vi "模拟反馈.vi"(0 "拆分信息-数据":T2, 5 "寄存器输入":u16[](array[numeric])) -> (14 "反馈参数":T1, 19 "寄存器输出":u16[](array[numeric]))   [LabVIEW 2019, in "MainPage.lvlib" / "MainPage.lvclass"]
uses:
  MainPage.lvclass
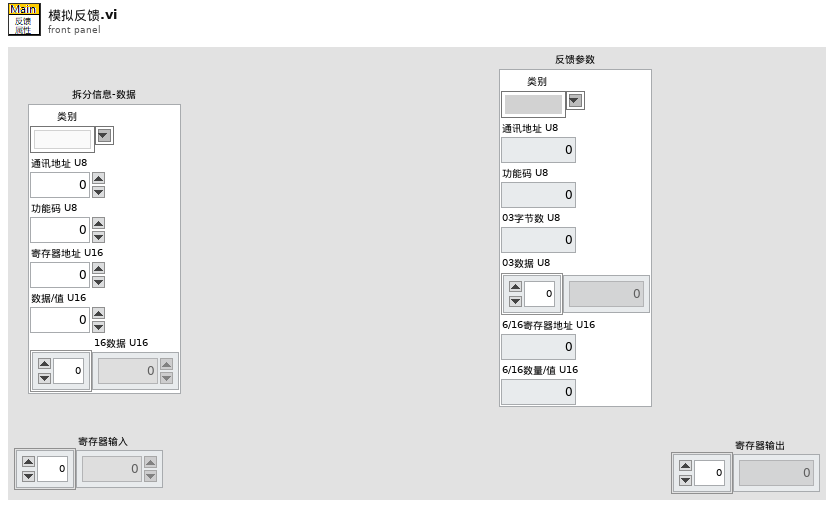
[diagram p1: front panel]
types:
  T1 = cluster{"类别":string, "通讯地址 U8":u8, "功能码 U8":u8, "03字节数 U8":u8, "03数据 U8":u8[], "6/16寄存器地址 U16":u16, "6/16数量/值 U16":u16}
  T2 = cluster{"类别":string, "通讯地址 U8":u8, "功能码 U8":u8, "寄存器地址 U16":u16, "数据/值 U16":u16, "16数据 U16":u16[]}
  T3 = cluster{"类别":string, "通讯地址 U8":u8, "功能码 U8":u8, u8, u8[], "寄存器地址 U16":u16, "数据/值 U16":u16}
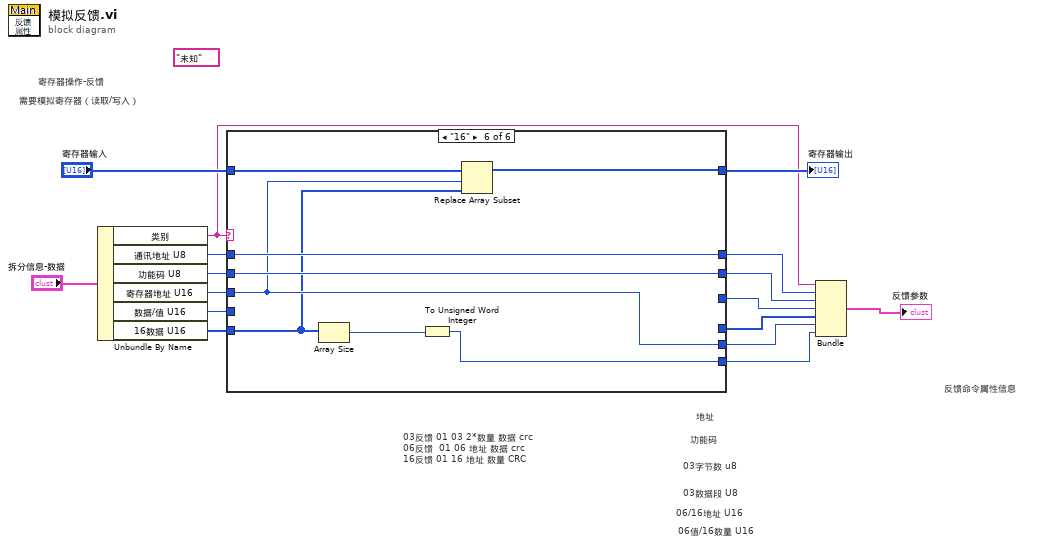
[diagram p0: block diagram]
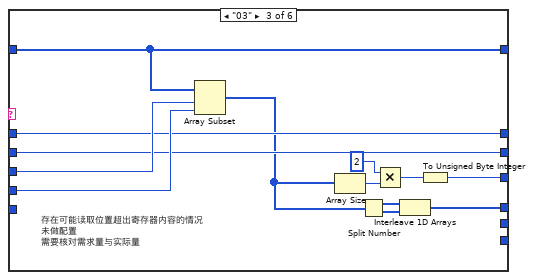
[diagram p4: hidden frame]
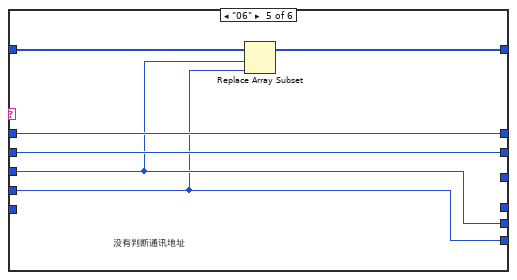
[diagram p6: hidden frame]
diagram:
  (unwired) "未知" ("类别")
  # "06值/16数量 U16"
  # "06/16地址 U16"
  # "03数据段 U8"
  # "03字节数 u8"
  # "功能码"
  # "地址"
  # "03反馈 01 03 2*数量 数据 crc\n06反馈  01 06 地址 数据 crc\n16反馈 01 16 地址 数量 CRC"
  # "反馈命令属性信息"
  # "需要模拟寄存器（读取/写入）"
  # "寄存器操作-反馈"
  n1 = Unbundle By Name("拆分信息-数据") -> ("类别"=w1:string, "通讯地址 U8"=w13:u8, "功能码 U8"=w12:u8, "寄存器地址 U16"=w11:u16, "数据/值 U16"=w10:u16, "16数据 U16"=w9:u16[])
  n2 = case shown="\"16\"" w1 {
    tunnel: "寄存器输入" -> [w17 w18 w31 w32 w36 w46]
    tunnel: [w17 w18 w31 w32 w33 w45] -> w14
    tunnel: w13 -> [_ _ w28 _ w38 w44]
    tunnel: w12 -> [_ _ w27 _ w37 w43]
    tunnel: w11 -> [_ _ w30 _ w35 w41]
    tunnel: w10 -> [_ _ w29 _ w34 _]
    tunnel: w9 -> [_ _ _ _ _ w40]
    tunnel: [_ _ w28 _ w38 w44] -> w8
    tunnel: [_ _ w27 _ w37 w43] -> w7
    tunnel: [_ _ w20 _ _ _] -> w5
    tunnel: [_ _ w19 _ _ _] -> w6
    tunnel: [_ _ _ _ w35 w41] -> w4
    tunnel: [_ _ _ _ w34 w42] -> w3
    frame Default {
    }
    frame "未知" {
    }
    frame "03" {
      # "存在可能读取位置超出寄存器内容的情况\n未做配置\n需要核对需求量与实际量"
      n3 = Array Subset(array=w31, index=w30, length=w29) -> (w21:u16[])
      n4 = Array Size(array=w21) -> (size(s)=w26:i32)
      n5 = Split Number(x=w21) -> (hi(x)=w23:u8[], lo(x)=w22:u8[])
      n6 = Multiply(x=2, y=w26) -> (x*y=w24:i32)
      n7 = Interleave 1D Arrays(w23, w22) -> (w20:u8[])
      n8 = To Unsigned Byte Integer(number=w24) -> (unsigned 8bit integer=w19:u8)
    }
    frame "05" {
    }
    frame "06" {
      # "没有判断通讯地址"
      n9 = Replace Array Subset(array=w36, new element=w34, index=w35) -> (w33:u16[])
    }
    frame "16" {
      n10 = Array Size(array=w40) -> (size(s)=w39:i32)
      n11 = To Unsigned Word Integer(number=w39) -> (unsigned 16bit integer=w42:u16)
      n12 = Replace Array Subset(array=w46, new element=w40, index=w41) -> (w45:u16[])
    }
  }
  "寄存器输出" <- w14
  n13 = Bundle("类别"=w1, "通讯地址 U8"=w8, "功能码 U8"=w7, w6, w5, "寄存器地址 U16"=w4, "数据/值 U16"=w3) -> (→"反馈参数":T3)  [unwired: 1 in]
